vi "CAN Communication.vi"(8 "error in":errorcluster) -> (0 "error out":errorcluster)   [LabVIEW 2016]
uses:
  Typedefs/CAN Refnum.ctl
  Typedefs/CAN Session Pointer.ctl
  Typedefs/CAN Communication References.ctl
  Typedefs/kill process notifier array.ctl
  Typedefs/Write Queue.ctl
  Typedefs/FPGA CAN Frame Cluster.ctl
  <vilib>/userdefined/High Color/nirio_resource_hc.ctl
  <vilib>/FPGAPlugInAG/cRIO-9033/niLvFpga_Open_cRIO-9033.vi
  <vilib>/Utility/error.llb/Error Cluster From Error Code.vi
  <vilib>/RVI Host/nirviSupport.llb/nirviErrorClusterFromErrorCode.vi
  <vilib>/rvi/errors/niLvFpgaAdjustHostInterfaceError.vi
  <vilib>/FPGAPlugInAG/cRIO-9033/niLvFpga_Close_cRIO-9033.vi
  <vilib>/rvi/interface/nirviOpenFPGA/nirviOpenFPGA.xnode
  Users/s163601/Desktop/05-28/FPGA Bitfiles/project_FPGATarget_FPGAMain_boaNRF5GBP4.lvbitx
  Users/s163601/Desktop/05-28/FPGA Main.vi
  <vilib>/rvi/interface/nirviMethod/nirviMethod.xnode
  <vilib>/rvi/interface/nirviReadWriteControl/nirviReadWriteControl.xnode
  <vilib>/rvi/interface/nirviCloseFPGA/nirviCloseFPGA.xnode
  NiFpgaLv.dll
  <vilib>/rvi/interface/nirviMethod/StockFPGA_InlinedMethodWaitForSingleIRQ.vi
  <vilib>/FPGAPlugInAG/cRIO-9033/niLvFpga_WaitOnIrq_cRIO-9033.vi
  <vilib>/FPGAPlugInAG/cRIO-9033/niLvFpga_AcknowledgeIrq_cRIO-9033.vi
panel:
  out "CAN Session Out":T1
  in  "CAN Session In":T1
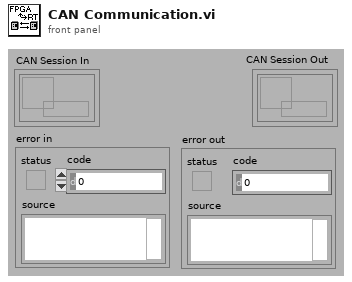
[diagram p1: front panel]
types:
  T1 = typedef "CAN Refnum.ctl" = refnum<k1>
  T2 = typedef "nirio_resource_hc.ctl" = tag
  T3 = typedef "kill process notifier array.ctl" = refnum<notifier>[]
  T4 = typedef "Write Queue.ctl" = refnum<queue>
  T5 = typedef "CAN Session Pointer.ctl" = refnum<queue>
  T6 = cluster{"Timestamp":u64, "Identifier":u32, "Type":u8, "InfoA":u8, "InfoB":u8, "DataLength":u8, "Data":u8[]}
  T7 = typedef "CAN Communication References.ctl" = cluster{"kill process notifier array":T3, "Write Queue":T4, "New Frame Notifier":refnum<notifier>, "Read Queue Array":T4[]}
  T8 = typedef "FPGA CAN Frame Cluster.ctl" = cluster{"Timestamp":u64, "Identifier":u32, "Type":u8, "InfoA":u8, "InfoB":u8, "DataLength":u8, "Data":u8[]}
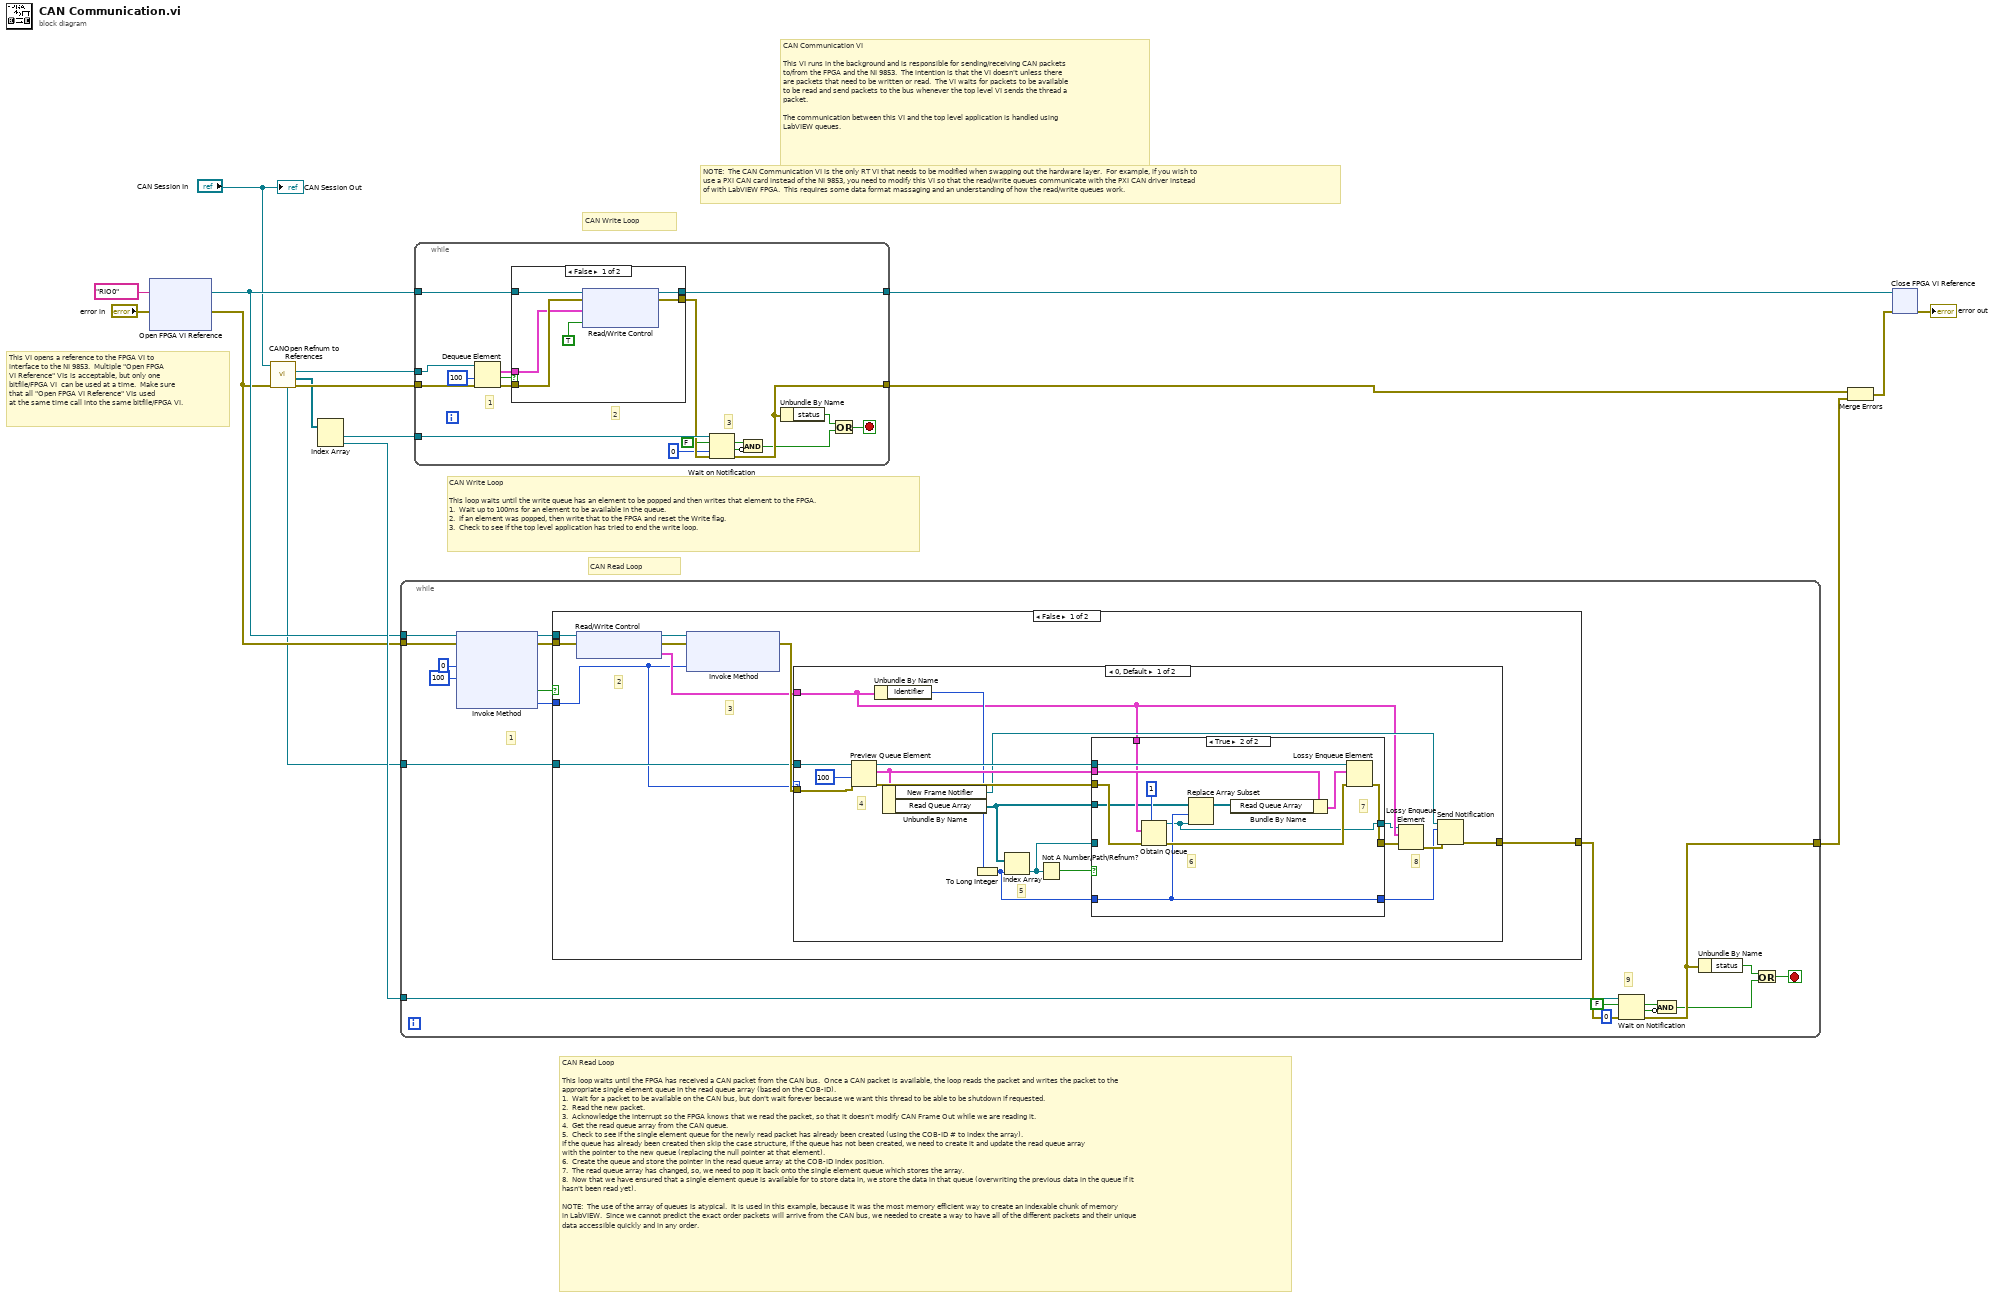
[diagram p0: block diagram]
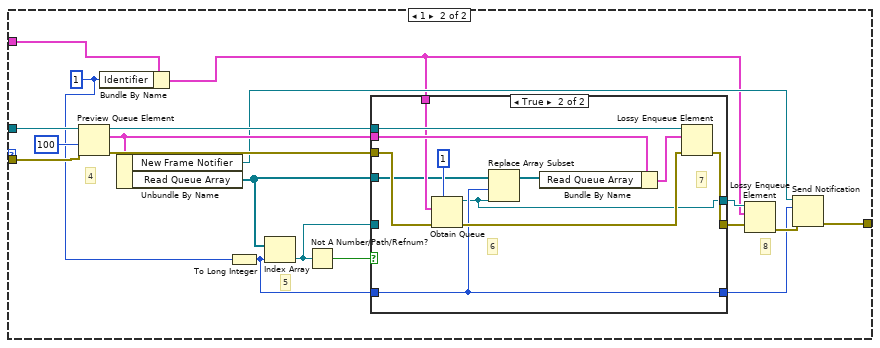
[diagram p4: hidden frame]
diagram:
  # "This VI opens a reference to the FPGA VI to\ninterface to the NI 9853.  Multiple \"Open FPGA\nVI Reference\" VIs is acceptable, but only one\nbitfile/FPGA VI  can be used at a time.  Make sure\nthat all \"Open FPGA VI Reference\" VIs used\nat the same time call into the same bitfile/FPGA VI."
  # "NOTE:  The CAN Communication VI is the only RT VI that needs to be modified when swapping out the hardware layer.  For example, if you wish to\nuse a PXI CAN card instead of the NI 9853, you need to modify this VI so that the read/write queues communicate with the PXI CAN driver instead\nof with LabVIEW FPGA.  This requires some data format massaging and an understanding of how the read/write queues work."
  # "CAN Read Loop\n\nThis loop waits until the FPGA has received a CAN packet from the CAN bus.  Once a CAN packet is available, the loop reads the packet and writes the packet to the\nappropriate single element queue in the read queue array (based on the COB-ID).\n1.  Wait for a packet to be available on the CAN bus, but don't wait forever because we want this thread to be able to be shutdown if requested.\n2.  Read the new packet.\n3.  Acknowledge the interrupt so the FPGA knows that we read the packet, so that it doesn't modify CAN Frame Out while we are reading it.\n4.  Get the read queue array from the CAN queue.\n5.  Check to see if the single element queue for the newly read packet has already been created (using the COB-ID # to index the array).\nIf the queue has already been created then skip the case structure, if the queue has not been created, we need to create it and update the read queue array\nwith the pointer to the new queue (replacing the null pointer at that element).\n6.  Create the queue and store the pointer in the read queue array at the COB-ID index position.\n7.  The read queue array has changed, so, we need to pop it back onto the single element queue which stores the array.\n8.  Now that we have ensured that a single element queue is available for to store data in, we store the data in that queue (overwriting the previous data in the queue if it\nhasn't been read yet).\n\nNOTE:  The use of the array of queues is atypical.  It is used in this example, because it was the most memory efficient way to create an indexable chunk of memory\nin LabVIEW.  Since we cannot predict the exact order packets will arrive from the CAN bus, we needed to create a way to have all of the different packets and their unique\ndata accessible quickly and in any order."
  # "CAN Write Loop\n\nThis loop waits until the write queue has an element to be popped and then writes that element to the FPGA.\n1.  Wait up to 100ms for an element to be available in the queue.\n2.  If an element was popped, then write that to the FPGA and reset the Write flag.\n3.  Check to see if the top level application has tried to end the write loop."
  # "CAN Communication VI\n\nThis VI runs in the background and is responsible for sending/receiving CAN packets\nto/from the FPGA and the NI 9853.  The intention is that the VI doesn't unless there\nare packets that need to be written or read.  The VI waits for packets to be available\nto be read and send packets to the bus whenever the top level VI sends the thread a\npacket.\n\nThe communication between this VI and the top level application is handled using\nLabVIEW queues."
  # "CAN Read Loop"
  # "CAN Write Loop"
  n1 = xnode "Open FPGA VI Reference"("error in"="error in", "resource name"=T2 "RIO0") -> ("FPGA VI Reference Out"=w9:refnum<k20>, "error out"=w7:errorcluster)
  n2 = call "CANOpen Refnum to References.vi"("error in (no error)"=w7, "CAN Session In"="CAN Session In") -> ("error out"=w16:errorcluster, "kill process notifier array"=w13:T3, "Write Queue"=w15:T4, "CAN Session Queue"=w1:T5)  [unwired: 6 out]
  n3 = Index Array(array=w13) -> (element #1=w14:refnum<notifier>, element #2=w12:refnum<notifier>)  [unwired: 2 in]
  n4 = while {
    tunnel: w9 -> [w25]
    tunnel: w7 -> [w24]
    tunnel: [w32] -> w10
    tunnel: w12 -> [w28]
    tunnel: w1 -> [w17]
    stop <- w35 stop-if-true
    # "9"
    # "1"
    n5 = xnode "Invoke Method"("FPGA VI Reference In"=w25, "error in"=w24, "IRQ Number(s)"=0, "Timeout (ms)"=100) -> ("FPGA VI Reference Out"=w21:refnum<k20>, "error out"=w20:errorcluster, "Timed Out"=w19:bool, "IRQ(s) Asserted"=w18:i32)
    n6 = case shown="False" w19 {
      tunnel: w20 -> [w43 w112]
      tunnel: [w38 w112] -> w33
      tunnel: w21 -> [w44 _]
      tunnel: w18 -> [w36 _]
      tunnel: w17 -> [w39 _]
      frame False {
        # "3"
        # "2"
        n7 = xnode "Read/Write Control"("FPGA VI Reference In"=w44, "error in"=w43) -> ("FPGA VI Reference Out"=w42:refnum<k20>, "error out"=w41:errorcluster, "CAN Frame Out"=w37:T6)
        n8 = xnode "Invoke Method"("FPGA VI Reference In"=w42, "error in"=w41, "IRQ Number(s)"=w36) -> ("error out"=w40:errorcluster)  [unwired: 1 out]
        n9 = case shown="0, Default" w36 {
          tunnel: w40 -> [w56 w90]
          tunnel: w39 -> [w55 w89]
          tunnel: [w51 w85] -> w38
          tunnel: w37 -> [w49 w80]
          frame 0, Default {
            # "8"
            # "5"
            # "4"
            n10 = Preview Queue Element(queue=w55, timeout in ms (-1)=100, error in (no error)=w56) -> (queue out=w59:T5, element=w54:T7, error out=w60:errorcluster)  [unwired: 1 out]
            n11 = Unbundle By Name(w49) -> ("Identifier"=w50:u32)
            n12 = Unbundle By Name(w54) -> ("New Frame Notifier"=w53:refnum<notifier>, "Read Queue Array"=w45:T4[])
            n13 = To Long Integer(number=w50) -> (32bit integer=w57:i32)
            n14 = Index Array(array=w45, index=w57) -> (element=w46:T4)
            n15 = Not A Number/Path/Refnum?(number/path/refnum=w46) -> (NaN/Path/Refnum?=w62:bool)
            n16 = case shown="True" w62 {
              tunnel: w57 -> [w64 w69]
              tunnel: [w63 w66] -> w47
              tunnel: w60 -> [w65 w71]
              tunnel: [w65 w75] -> w61
              tunnel: w59 -> [_ w72]
              tunnel: w54 -> [_ w73]
              tunnel: w46 -> [w63 _]
              tunnel: w49 -> [_ w70]
              tunnel: [w64 w69] -> w48
              tunnel: w45 -> [_ w67]
              frame False {
              }
              frame True {
                # "7"
                # "6"
                n17 = Obtain Queue(max queue size (-1, unlimited)=1, element data type=w70, error in (no error)=w71) -> (queue out=w66:refnum<queue>, error out=w74:errorcluster)  [unwired: 1 in, 2 out]
                n18 = Replace Array Subset(array=w67, new element=w66, index=w69) -> (w68:T4[])
                n19 = Bundle By Name(cluster=w73, "Read Queue Array"=w68) -> (w76:T7)
                n20 = Lossy Enqueue Element(queue=w72, element=w76, error in (no error)=w74) -> (error out=w75:errorcluster)  [unwired: 3 out]
              }
            }
            n21 = Lossy Enqueue Element(queue=w47, element=w49, error in (no error)=w61) -> (error out=w52:errorcluster)  [unwired: 3 out]
            n22 = Send Notification(notification=w48, notifier=w53, error in (no error)=w52) -> (error out=w51:errorcluster)  [unwired: 1 out]
          }
          frame 1 {
            w78 = u32 1 ("Identifier")
            # "8"
            # "5"
            # "4"
            n23 = Preview Queue Element(queue=w89, timeout in ms (-1)=100, error in (no error)=w90) -> (queue out=w93:T5, element=w88:T7, error out=w94:errorcluster)  [unwired: 1 out]
            n24 = Bundle By Name(cluster=w80, "Identifier"=w78) -> (w79:T6)
            n25 = Unbundle By Name(w88) -> ("New Frame Notifier"=w87:refnum<notifier>, "Read Queue Array"=w81:T4[])
            n26 = To Long Integer(number=w78) -> (32bit integer=w91:i32)
            n27 = Index Array(array=w81, index=w91) -> (element=w82:T4)
            n28 = Not A Number/Path/Refnum?(number/path/refnum=w82) -> (NaN/Path/Refnum?=w96:bool)
            n29 = case shown="True" w96 {
              tunnel: w91 -> [w98 w103]
              tunnel: [w97 w100] -> w83
              tunnel: w94 -> [w99 w105]
              tunnel: [w99 w109] -> w95
              tunnel: w93 -> [_ w106]
              tunnel: w88 -> [_ w107]
              tunnel: w82 -> [w97 _]
              tunnel: w79 -> [_ w104]
              tunnel: [w98 w103] -> w84
              tunnel: w81 -> [_ w101]
              frame False {
              }
              frame True {
                # "7"
                # "6"
                n30 = Obtain Queue(max queue size (-1, unlimited)=1, element data type=w104, error in (no error)=w105) -> (queue out=w100:refnum<queue>, error out=w108:errorcluster)  [unwired: 1 in, 2 out]
                n31 = Replace Array Subset(array=w101, new element=w100, index=w103) -> (w102:T4[])
                n32 = Bundle By Name(cluster=w107, "Read Queue Array"=w102) -> (w110:T7)
                n33 = Lossy Enqueue Element(queue=w106, element=w110, error in (no error)=w108) -> (error out=w109:errorcluster)  [unwired: 3 out]
              }
            }
            n34 = Lossy Enqueue Element(queue=w83, element=w79, error in (no error)=w95) -> (error out=w86:errorcluster)  [unwired: 3 out]
            n35 = Send Notification(notification=w84, notifier=w87, error in (no error)=w86) -> (error out=w85:errorcluster)  [unwired: 1 out]
          }
        }
      }
      frame True {
      }
    }
    n36 = Wait on Notification(notifier=w28, ignore previous (F)=FALSE, timeout in ms (-1)=0, error in (no error)=w33) -> (notification=w31:bool, timed out?=w30:bool, error out=w32:errorcluster)  [unwired: 1 out]
    n37 = Compound Arithmetic op=AND(w31, invert w30) -> (w29:bool)
    n38 = Unbundle By Name(w32) -> ("status"=w34:bool)
    n39 = Or(x=w34, y=w29) -> (x .or. y?=w35:bool)
  }
  n40 = while {
    tunnel: w9 -> [w130]
    tunnel: [w119] -> w11
    tunnel: w16 -> [w127]
    tunnel: w15 -> [w122]
    tunnel: w14 -> [w121]
    tunnel: [w113] -> w6
    stop <- w129 stop-if-true
    # "3"
    # "2"
    # "1"
    n41 = Dequeue Element(queue=w122, timeout in ms (-1)=100, error in (no error)=w127) -> (element=w126:T8, timed out?=w123:bool, error out=w125:errorcluster)  [unwired: 1 out]
    n42 = case shown="False" w123 {
      tunnel: w130 -> [w135 w137]
      tunnel: [w134 w138] -> w120
      tunnel: w126 -> [w132 _]
      tunnel: w125 -> [w136 w138]
      tunnel: [w131 w137] -> w113
      frame False {
        n43 = xnode "Read/Write Control"("FPGA VI Reference In"=w135, "error in"=w136, "CAN Frame In"=w132, "Write"=TRUE) -> ("FPGA VI Reference Out"=w131:refnum<k20>, "error out"=w134:errorcluster)
      }
      frame True {
      }
    }
    n44 = Wait on Notification(notifier=w121, ignore previous (F)=FALSE, timeout in ms (-1)=0, error in (no error)=w120) -> (notification=w116:bool, timed out?=w115:bool, error out=w119:errorcluster)  [unwired: 1 out]
    n45 = Compound Arithmetic op=AND(w116, invert w115) -> (w114:bool)
    n46 = Unbundle By Name(w119) -> ("status"=w128:bool)
    n47 = Or(x=w128, y=w114) -> (x .or. y?=w129:bool)
  }
  n48 = Merge Errors(w11, w10) -> (w5:errorcluster)
  n49 = xnode "Close FPGA VI Reference"("FPGA VI Reference In"=w6, "error in"=w5) -> ("error out"=→"error out":errorcluster)
  "CAN Session Out" <- "CAN Session In"
